vi "PSTR-Start AO.vi"(0 "Runtime":T1 {"window" items=["None ", "Hanning", "Hamming", "Blackman-Harris", "Exact Blackman", "Blackman", "Flat Top", "4 Term B-Harris ", "7 Term B-Harris", "Low Sidelobe"]}) -> (4 "Runtime out":T1 {"window" items=["None ", "Hanning", "Hamming", "Blackman-Harris", "Exact Blackman", "Blackman", "Flat Top", "4 Term B-Harris ", "7 Term B-Harris", "Low Sidelobe"]}, 15 "error out":errorcluster)   [LabVIEW 2020]
uses:
  Typedefs/PSTR-Runtime Data.ctl
  epl-vi-lib/Signal Synthesis VIs/4th Generation/Classes/SignalManager/SignalManager.lvclass
  epl-vi-lib/PXI DAQ VIs/AODO/Typedefs/AODO-Action.ctl
  epl-vi-lib/Signal Synthesis VIs/4th Generation/Classes/SignalManager/SignalManager.lvclass/SignalManager.ctl
  epl-vi-lib/Signal Synthesis VIs/4th Generation/Classes/Channel/Channel.lvclass/Channel.ctl
  epl-vi-lib/Signal Synthesis VIs/4th Generation/Classes/Level/Level.lvclass/Level.ctl
  epl-vi-lib/Signal Synthesis VIs/4th Generation/Classes/Channel/Write Level Value.vi
  epl-vi-lib/Signal Synthesis VIs/4th Generation/Classes/Level/Write Level.vi
  epl-vi-lib/Signal Synthesis VIs/4th Generation/Classes/Channel/Channel.lvclass
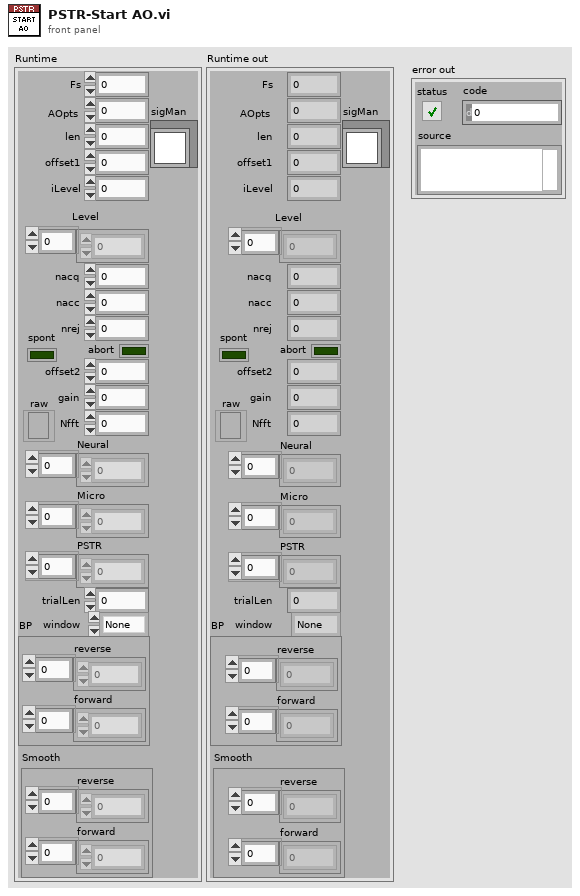
[diagram p1: front panel]
types:
  T1 = typedef "PSTR-Runtime Data.ctl" = cluster{"Fs":dbl, "AOpts":i32, "len":i32, "offset1":i32, "iLevel":i32, "Level":dbl[], "nacc":i32, "nrej":i32, "nacq":i32, "abort":bool, "offset2":i32, "gain":dbl, "Nfft":i32, "Neural":dbl[], "Micro":dbl[], "raw":refnum<file>, "spont":bool, "PSTR":dbl[], "trialLen":i32, "window":u16, "BP":cluster{"reverse":dbl[], "forward":dbl[]}, "Smooth":cluster{"reverse":dbl[], "forward":dbl[]}, "sigMan":refnum<class "SignalManager.lvclass">}
  T2 = typedef "AODO-Action.ctl" = enum16{"Configure", "Initialize", "Start", "Write", "Clean up", "Init & Start", "Config & Test", "Position", "Set AO Gains", "Zero", "Prime", "Status"}
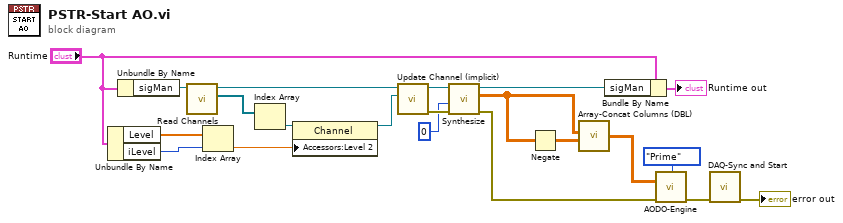
[diagram p0: block diagram]
diagram:
  n1 = Unbundle By Name("Runtime") -> ("Level"=w19:dbl[], "iLevel"=w18:i32)
  n2 = Unbundle By Name("Runtime") -> ("sigMan"=w20:refnum<class "SignalManager.lvclass">)
  n3 = call "Read Channels.vi"("SignalManager in"=w20) -> ("Channels"=w17:refnum<class "Channel.lvclass">[], "SignalManager out"=w14:refnum<class "SignalManager.lvclass">)  [unwired: 8 in, 1 out]
  n4 = Index Array(array=w19, index=w18) -> (element=w15:dbl)
  n5 = Index Array(array=w17) -> (element=w16:refnum<class "Channel.lvclass">)  [unwired: 1 in]
  n6 = property class="Channel"(reference=w16, "Accessors:Level 2"=w15) -> (reference out=w13:refnum<class "Channel.lvclass">)  [unwired: 1 in, 1 out]
  n7 = call "Update Channel (implicit).vi"("Channel"=w13, "SignalManager in"=w14) -> ("error out"=w5:errorcluster, "SignalManager out"=w12:refnum<class "SignalManager.lvclass">)  [unwired: 8 in]
  n8 = call "Synthesize.vi"("error in (no error)"=w5, "Repetition"=0, "SigMan in"=w12) -> ("error out"=w11:errorcluster, "Array"=w3:dbl[][], "SigMan out"=w7:refnum<class "SignalManager.lvclass">)  [unwired: 6 in]
  n9 = Negate(x=w3) -> (-x=w2:dbl[][])
  n10 = call "Array-Concat Columns (DBL).vi"("Array 2"=w2, "Array 1"=w3) -> ("concatenated array"=w1:dbl[][])  [unwired: 4 in]
  n11 = Bundle By Name(cluster="Runtime", "sigMan"=w7) -> (→"Runtime out":T1)
  n12 = call "AODO-Engine.vi"("Action"=AODO-Action."Prime", "AO"=w1, "error in (no error)"=w11) -> ("error out"=w9:errorcluster)  [unwired: 7 in, 5 out]
  n13 = call "DAQ-Sync and Start.vi"("error in (no error)"=w9) -> ("error out"=→"error out":errorcluster)  [unwired: 14 in]
